vi "Transfer External To Ext Or Ext10.vi"(4 "Trigger Level 2":dbl, 6 "Trigger Level":dbl, 8 "error in (no error)":errorcluster, 10 "Trigger Source With External":u16, 11 "VISA resource name":refnum<visa-resource-name>) -> (0 "error out":errorcluster, 2 "Trigger Source With Ext/Ext10":u16, 3 "VISA resource name out":refnum<visa-resource-name>)   [LabVIEW 2015, in "LeCroy Wave Series.lvlib"]
doc: "This is function which transfer Eternal trigger source to Ext and Ext10. Another trigger source are retained in same state. Transfer External source to Ext and Ext10 is make with compare trigger level. When is trigger level greater than 400 mV (for WaveSurfer 500 mV), than External trigger source is transfer to the Ext10, else is transfer to the Ext."
uses:
  <instrlib>/LeCroy Wave Series/LeCroy Wave Series.lvlib
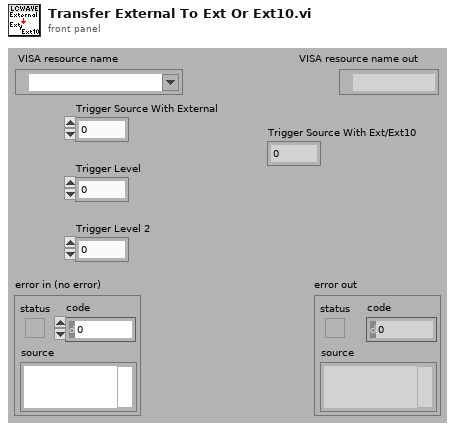
[diagram p1: front panel]
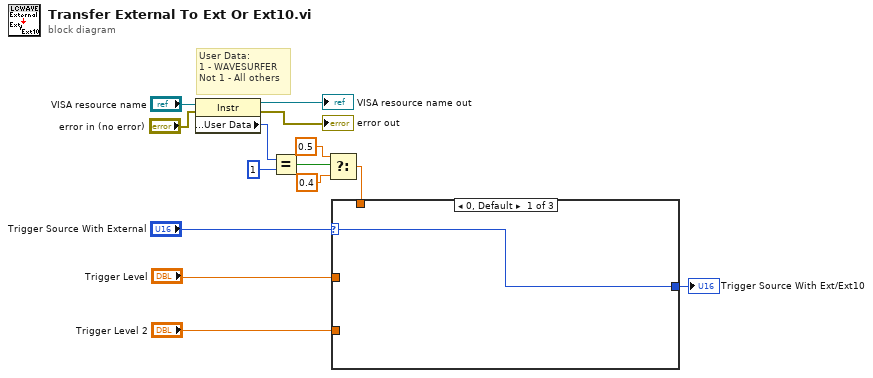
[diagram p0: block diagram]
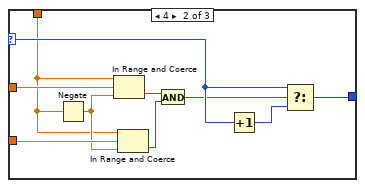
[diagram p2: hidden frame]
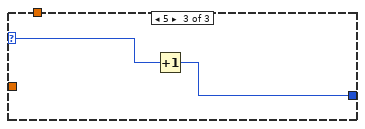
[diagram p3: hidden frame]
diagram:
  # "User Data:\n1 - WAVESURFER\nNot 1 - All others"
  n1 = property on="Property Node" class="Instr"(reference="VISA resource name", error in="error in (no error)") -> (reference out=→"VISA resource name out":refnum<visa-resource-name>, error out=→"error out":errorcluster, "General Settings:User Data"=w6:u32)
  n2 = Equal?(x=w6, y=u32 1) -> (x = y?=w4:bool)
  n3 = Select(t=0.5 ("upper limit"), s=w4, f=0.4 ("upper limit")) -> (s? t:f=w3:dbl)
  n4 = case shown="0, Default" "Trigger Source With External" {
    selector: "Trigger Source With External" -> [w15 w24 w27]
    tunnel: [w15 w22 w26] -> w12
    tunnel: "Trigger Level" -> [_ w25 _]
    tunnel: "Trigger Level 2" -> [_ w21 _]
    tunnel: w3 -> [_ w16 _]
    frame 0, Default {
    }
    frame 4 {
      n5 = Negate(x=w16) -> (-x=w17:dbl)
      n6 = In Range and Coerce(upper limit=w16, x=w25, lower limit=w17) -> (In Range?=w20:bool)  [unwired: 1 out]
      n7 = In Range and Coerce(upper limit=w16, x=w21, lower limit=w17) -> (In Range?=w19:bool)  [unwired: 1 out]
      n8 = And(x=w20, y=w19) -> (x .and. y?=w18:bool)
      n9 = Increment(x=w24) -> (x+1=w23:u16)
      n10 = Select(t=w24, s=w18, f=w23) -> (s? t:f=w22:u16)
    }
    frame 5 {
      n11 = Increment(x=w27) -> (x+1=w26:u16)
    }
  }
  "Trigger Source With Ext/Ext10" <- w12
